vi "grSim_Replacement.vi"(5 "grSim_RobotReplacement":T1[](array[typedef]), 11 "grSim_BallReplacement":T2) -> (1 "Array":u8[](array[numeric]))   [LabVIEW 2016]
uses:
  grSim_BallReplacement.ctl
  grSim RobotReplacement.ctl
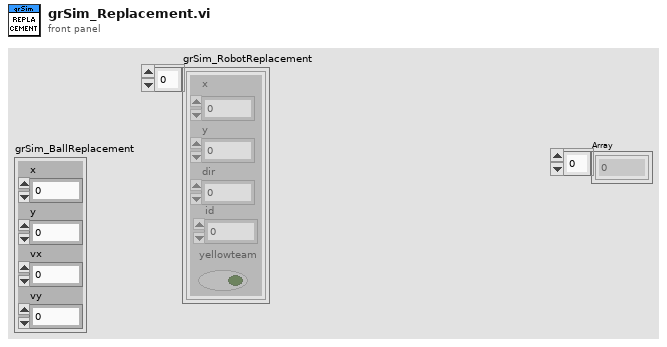
[diagram p1: front panel]
types:
  T1 = typedef "grSim RobotReplacement.ctl" = cluster{"x":dbl, "y":dbl, "dir":dbl, "yellowteam":bool, "id":u32}
  T2 = typedef "grSim_BallReplacement.ctl" = cluster{"x":dbl, "y":dbl, "vx":dbl, "vy":dbl}
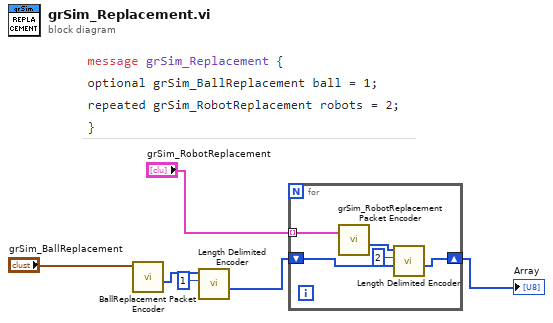
[diagram p0: block diagram]
diagram:
  n1 = call "BallReplacement Packet Encoder.vi"("grSim_BallReplacement"="grSim_BallReplacement") -> ("Array"=w5:u8[])  [unwired: 10 in]
  n2 = call "Length Delimited Encoder.vi"("Key"=u32 1, "Array In 2"=w5) -> ("Array"=w2:u8[])  [unwired: 9 in]
  n3 = for {
    tunnel: "grSim_RobotReplacement" -> [w11] mode=indexing
    shift-right: [w9] -> w1
    shift-left: w2 -> [w10]
    n4 = call "grSim_RobotReplacement Packet Encoder.vi"("grSim_RobotReplacement"=w11) -> ("Array"=w8:u8[])  [unwired: 10 in]
    n5 = call "Length Delimited Encoder.vi"("Array In"=w10, "Key"=u32 2, "Array In 2"=w8) -> ("Array"=w9:u8[])  [unwired: 8 in]
  }
  "Array" <- w1
